vi "Compass Init.vi"(6 "error in (no error)":errorcluster, 9 "FPGA VI Reference":T2) -> (0 "error out":errorcluster, 3 "FPGA Information Out":T1)   [LabVIEW 2012, in "Compass IO.lvlib"]
uses:
  Compass IO.lvlib
  FPGA_ref.ctl
  <vilib>/IEDriver/SPIandI2C/Host/I2C/I2C Host.lvlib
panel:
  # "Compass I2C interface\n=====\nInitialize compass communication and set to Continuous Read @ 20Hz.\nHeading can then be read out using Compass Read block.\nDefault ettings below should work in all cases."
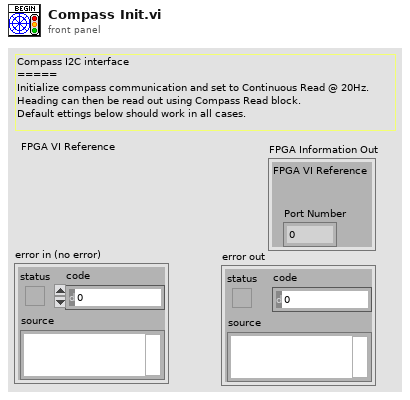
[diagram p1: front panel]
types:
  T1 = cluster{"FPGA VI Reference":refnum<k20>, "Port Number":u8}
  T2 = typedef "FPGA_ref.ctl" = refnum<k20>
  T3 = cluster{"FPGA VI Reference":T2, "Port Number":u8}
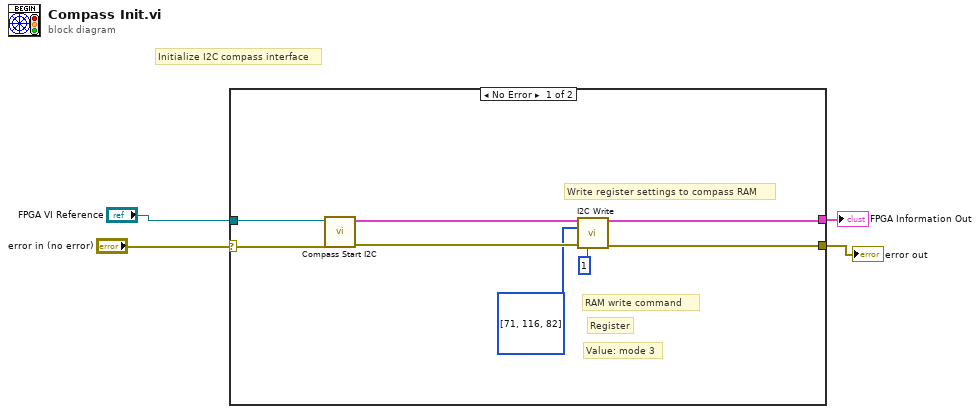
[diagram p0: block diagram]
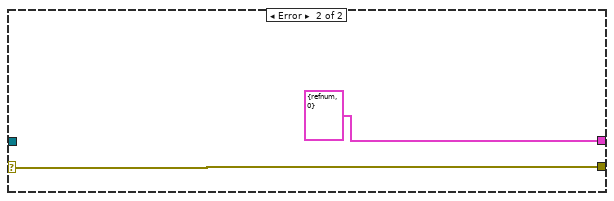
[diagram p2: hidden frame]
diagram:
  # "Initialize I2C compass interface"
  n1 = case shown="No Error" "error in (no error)" {
    selector: "error in (no error)" -> [w11 w14]
    tunnel: "FPGA VI Reference" -> [w12 _]
    tunnel: [w8 w14] -> w3
    tunnel: [w5 T3 {"FPGA VI Reference"=refnum, "Port Number"=0} ("FPGA Information Out")] -> w1
    frame No Error {
      # "Value: mode 3"
      # "Register"
      # "RAM write command"
      # "Write register settings to compass RAM"
      n2 = call "Compass Start I2C.vi"("error in (no error)"=w11, "Refnum in"=w12) -> ("error out"=w9:errorcluster, "FPGA Information Out"=w10:T1)  [unwired: 8 in]
      n3 = call <vilib>:"I2C Write.vi"("FPGA Information In"=w10, "Data"=u8[] [71, 116, 82], "error in (no error)"=w9, "Timeout (10 s)"=u8 1) -> ("FPGA Information Out"=w5:T1, "error out"=w8:errorcluster)  [unwired: 10 in]
    }
    frame Error {
    }
  }
  "error out" <- w3
  "FPGA Information Out" <- w1
